vi "configuration UI.vi"() -> ()   [LabVIEW 2014, in "Tagbus PID Module editor node.lvclass"]
uses:
  Tagbus PID Module editor node.lvclass
  module/configuration/Tagbus PID Module configuration.lvclass
  <vilib>/NI/Module Execution Interface/Engine Configuration/engine configuration.lvclass
  <vilib>/NI/Tag Bus Data Framework/Configuration Editor/Classes/Module editor node/module editor node.lvclass
  <vilib>/NI/Tag Bus Data Framework/Configuration Editor/Classes/Engine Parent/Engine Parent Editor Node.lvclass
  <vilib>/NI/Configuration Framework/serializable configuration/NISE_CEF_serializable configuration.lvclass
  <vilib>/NI/Tag Bus Module Framework/channel/TBM channel.lvclass
  <vilib>/NI/Tools/Keyed Array/KeyedArray.ctl
  <vilib>/NI/Tools/Keyed Array/Tools_KeyedArray.lvlib
  <vilib>/NI/AMC/Message.ctl
  <vilib>/NI/AMC/AMC.lvlib
  <vilib>/NI/AMC/Message Queue.ctl
  <vilib>/NI/Configuration Framework/Node/NISE_CEF_Node.lvclass
  <vilib>/NI/Configuration Framework/Node/NodeRef.ctl
  <vilib>/NI/Configuration Framework/Controls/EventCluster.ctl
  <vilib>/NI/Configuration Framework/NISE_CEF_TreeControl.lvlib
  <vilib>/NI/Configuration Framework/Node/UserEventRef.ctl
  <vilib>/NI/Configuration Framework/Node/StopEvent.ctl
  <vilib>/NI/Configuration Framework/Node/RefreshUIEvent.ctl
  <vilib>/NI/Configuration Framework/Node/CacheState.ctl
  <vilib>/NI/Configuration Framework/Node/NodeChangeEvent.ctl
panel:
  in  "node change":T1
  in  "cache state":T2
  in  "refresh UI":T3
  in  "stop event":T4
  in  "Tab Control":enum32{"Static Configuration"}(tab)
  in  "hidden_remove":bool
  in  "hidden_settings":bool
  in  "hidden_Add":bool
  in  "Remove Button":bool
  in  "Add Button":bool
  in  "channel":i32(listbox)
  in  "settings":bool
  in  "user event":T5
  in  "main queue":T6
  in  "node ref":T7
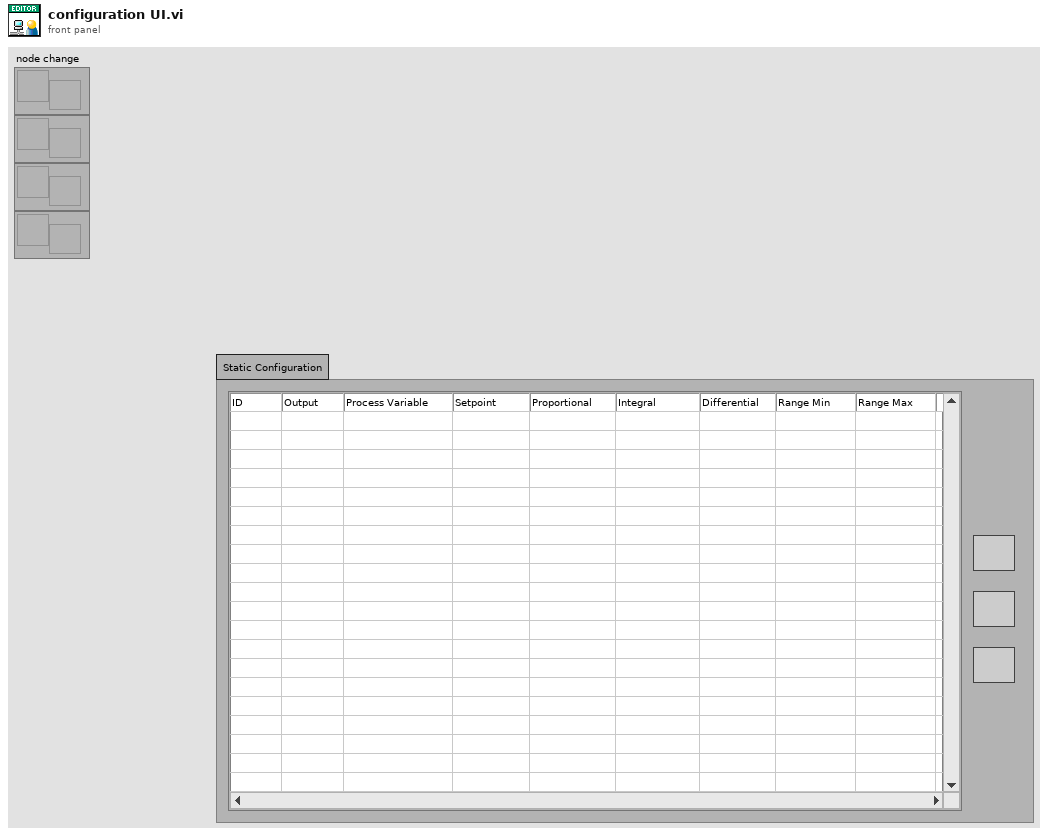
[diagram p1: front panel]
types:
  T1 = typedef "NISE_CEF_Node.lvclass/NodeChangeEvent.ctl" = refnum<user-event>
  T2 = typedef "NISE_CEF_Node.lvclass/CacheState.ctl" = refnum<user-event>
  T3 = typedef "NISE_CEF_Node.lvclass/RefreshUIEvent.ctl" = refnum<user-event>
  T4 = typedef "NISE_CEF_Node.lvclass/StopEvent.ctl" = refnum<user-event>
  T5 = typedef "NISE_CEF_Node.lvclass/UserEventRef.ctl" = refnum<user-event>
  T6 = typedef "AMC.lvlib/Message Queue.ctl" = refnum<queue>
  T7 = typedef "NISE_CEF_Node.lvclass/NodeRef.ctl" = refnum<data-value>
  T8 = typedef "Tagbus PID Module editor node.lvclass/table line.ctl" = cluster{"ID":string, "Setpoint":refnum<class "TBM channel.lvclass">, "Process Variable":refnum<class "TBM channel.lvclass">, "Output":refnum<class "TBM channel.lvclass">, "PID gains":cluster{"proportional gain (Kc)":dbl, "integral time (Ti, min)":dbl, "derivative time (Td, min)":dbl}, "output range":cluster{"output high":dbl, "output low":dbl}}
  T9 = cluster{"ID":string, "Setpoint":refnum<class "TBM channel.lvclass">, "Process Variable":refnum<class "TBM channel.lvclass">, "Output":refnum<class "TBM channel.lvclass">, "PID gains":cluster{"proportional gain (Kc)":dbl, "integral time (Ti, min)":dbl, "derivative time (Td, min)":dbl}, "output range":cluster{"output high":dbl, "output low":dbl}}
  T10 = typedef "LVPoint32TypeDef.ctl" = cluster{"Horizontal":i32, "Vertical":i32}
  T11 = typedef "LVRowAndColumnTypeDef.ctl" = cluster{"Row":i32, "Column":i32}
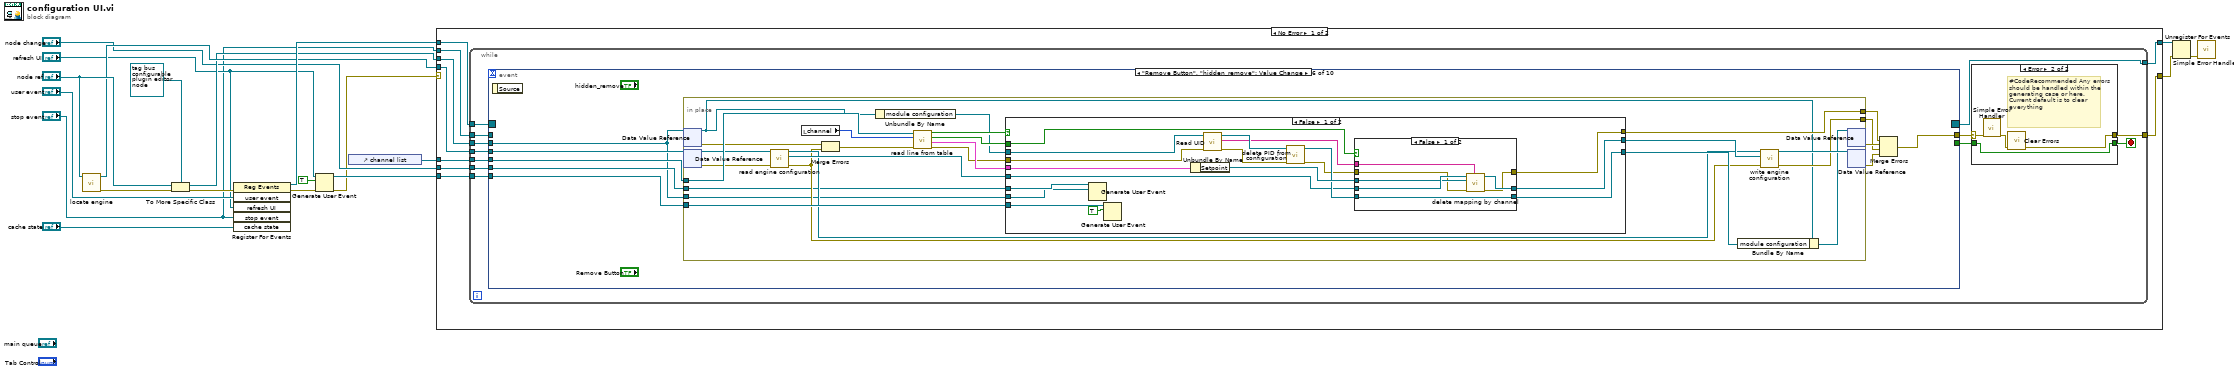
[diagram p0: block diagram]
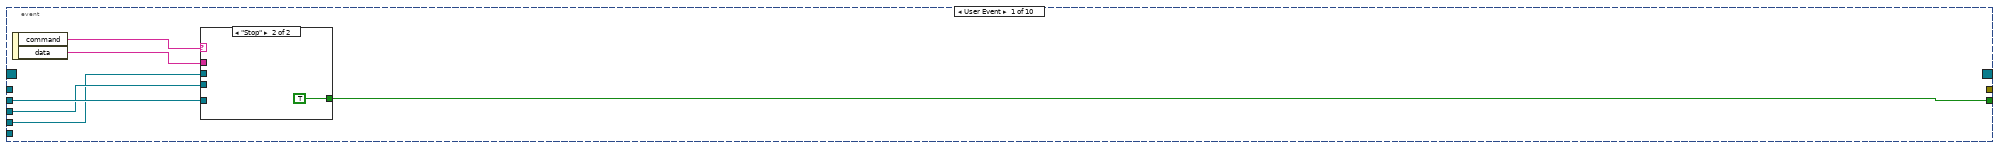
[diagram p3: hidden frame]
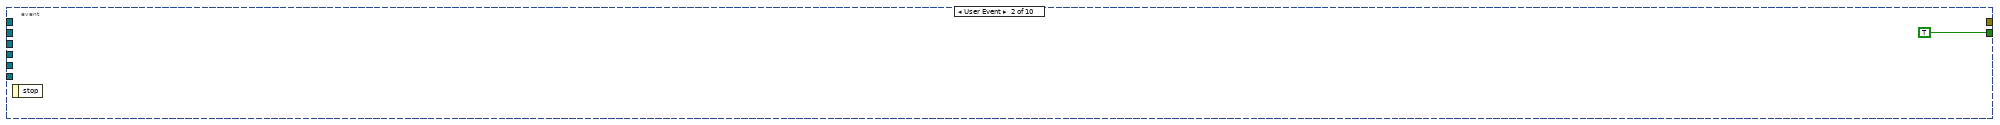
[diagram p5: hidden frame]
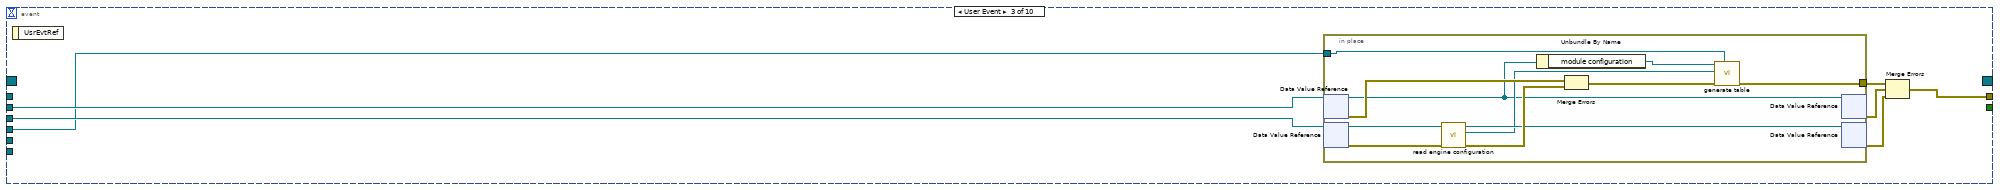
[diagram p6: hidden frame]
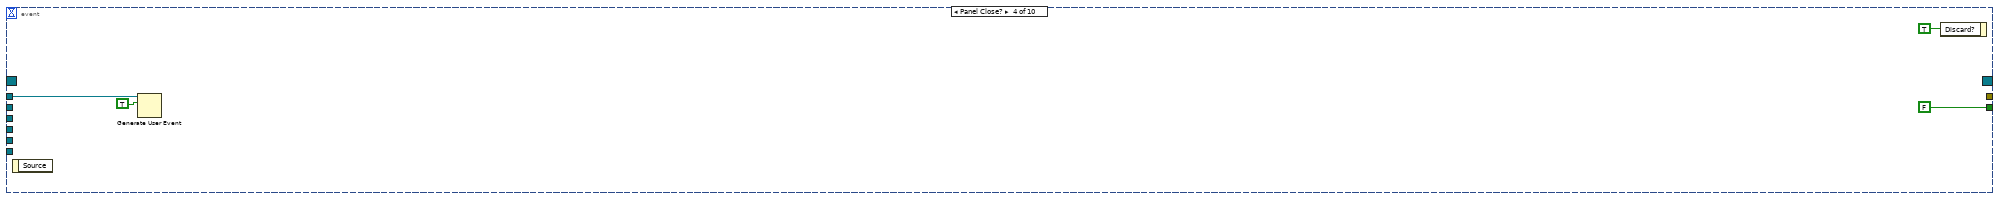
[diagram p7: hidden frame]
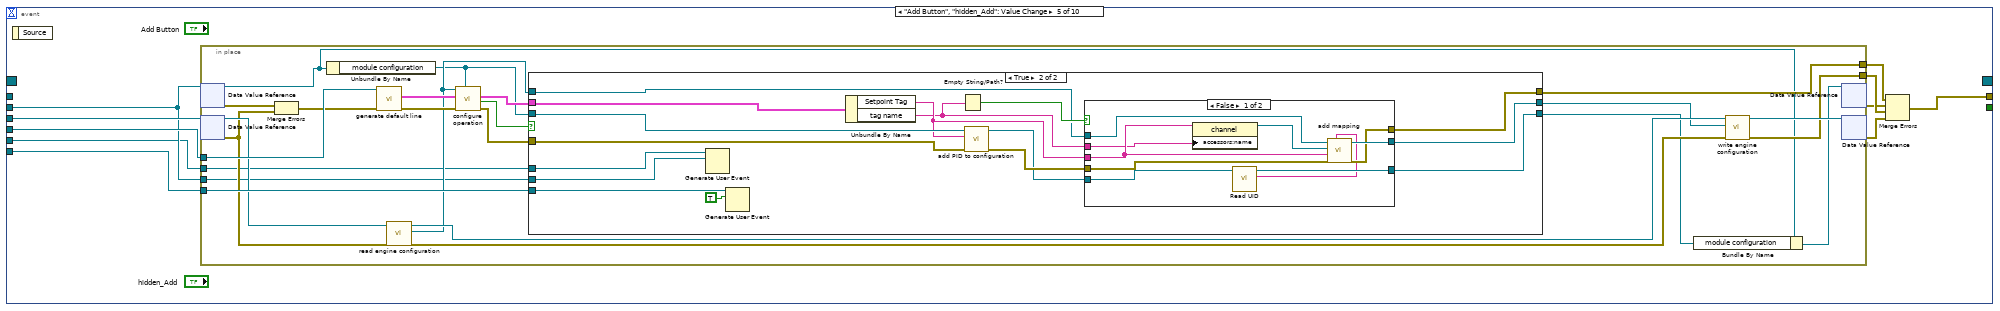
[diagram p8: hidden frame]
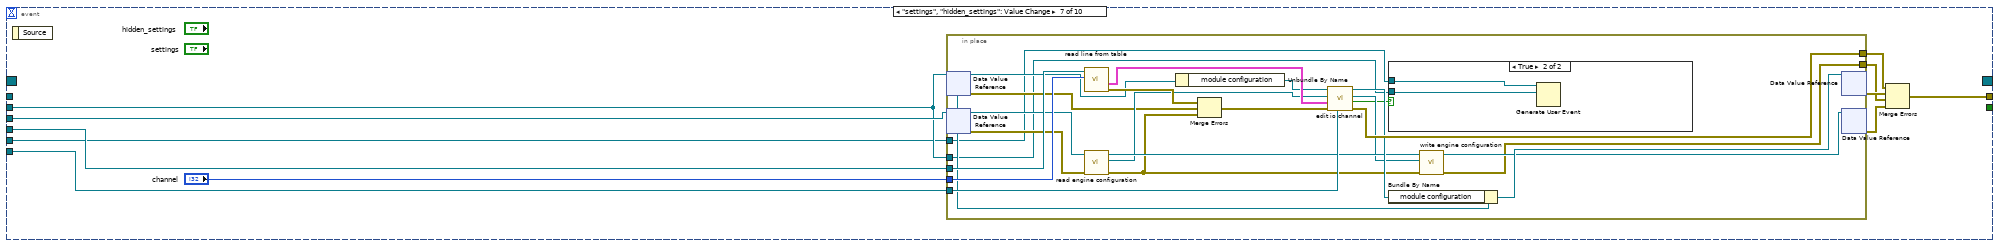
[diagram p13: hidden frame]
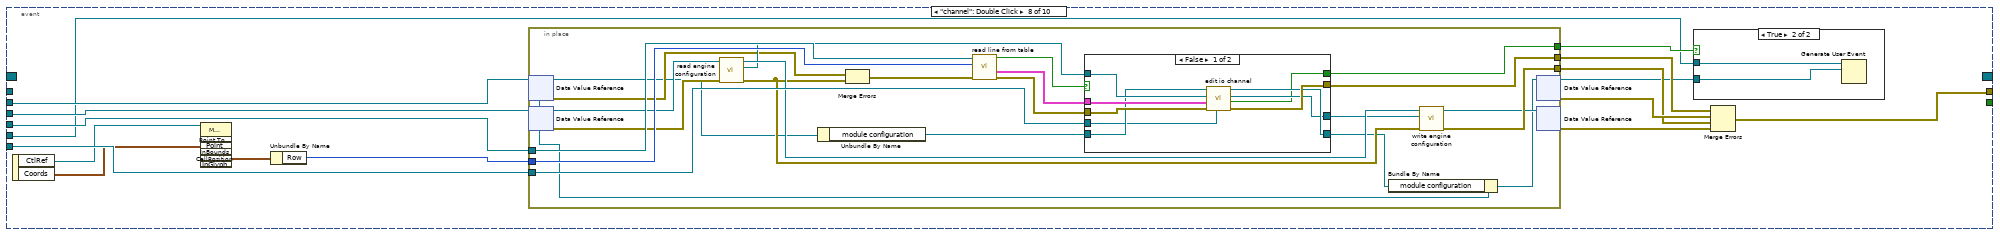
[diagram p15: hidden frame]
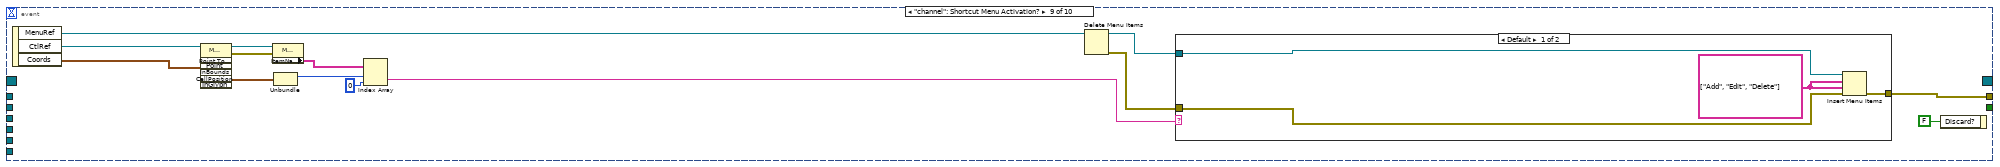
[diagram p18: hidden frame]
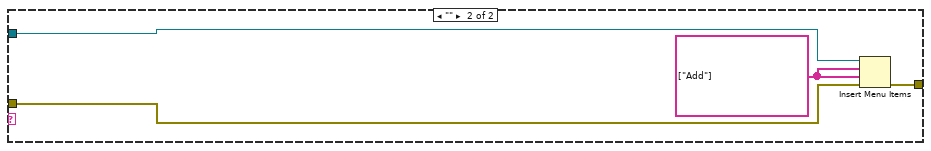
[diagram p19: hidden frame]
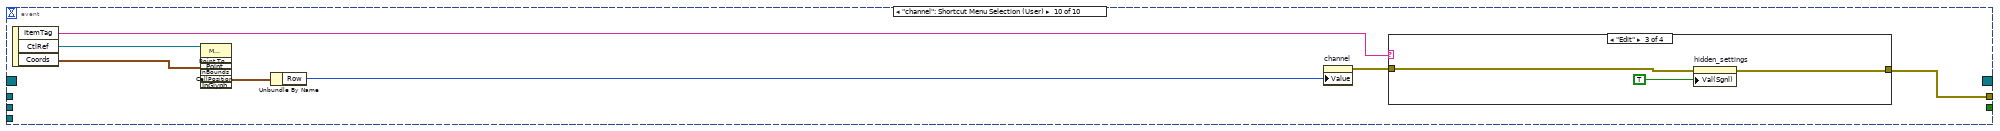
[diagram p20: hidden frame]
diagram:
  n1 = call <vilib>:"locate engine.vi"("component"="node ref") -> ("error out"=w8:errorcluster, "engine"=w15:refnum<data-value>)  [unwired: 9 in]
  n2 = To More Specific Class(target class=refnum<data-value> refnum ("data value reference"), reference="node ref", error in=w8) -> (specific class reference=w11:refnum<data-value>, error out=w10:errorcluster)
  n3 = register-events(error in=w10, "user event", "refresh UI", "stop event", "cache state") -> (reference out=w20:refnum<event-registration>, error out=w16:errorcluster)  [unwired: 1 in]
  n4 = Generate User Event(user event="refresh UI", event data cluster=TRUE ("event data"), error in=w16) -> (user event out=w7:T3, error out=w2:errorcluster)  [unwired: 1 in]
  n5 = control-ref of="channel list"() -> (w13:refnum<vi>)
  n6 = case shown="No Error" w2 {
    selector: w2 -> [_ w338]
    tunnel: w20 -> [w29 w337]
    tunnel: [w28 w337] -> w19
    tunnel: [w27 w338] -> w18
    tunnel: w15 -> [w26 _]
    tunnel: w13 -> [w25 _]
    tunnel: w11 -> [w24 _]
    tunnel: w7 -> [w23 _]
    tunnel: "node change" -> [w22 _]
    tunnel: "stop event" -> [w21 _]
    frame No Error {
      n7 = while {
        tunnel: w29 -> [w41]
        tunnel: [w40] -> w28
        tunnel: w24 -> [w36]
        tunnel: w26 -> [w35]
        tunnel: w23 -> [w34]
        tunnel: w25 -> [w32]
        tunnel: w22 -> [w31]
        tunnel: [w37] -> w27
        tunnel: w21 -> [w30]
        stop <- w39 stop-if-true
        n8 = event shown="[5] \"Remove Button\", \"hidden_remove\": Value Change" {
          selector: w41 -> [_ _ _ _ _ _ _ _ _ _]
          dyn-events: [_ _ _ _ _ _ _ _ _ _] -> w40
          timeout: _ -> [_ _ _ _ _ _ _ _ _ _]
          tunnel: [w53 TRUE _ FALSE _ _ _ _ _ _] -> w38
          tunnel: [_ _ w60 _ w84 w149 w216 w254 w298 w323] -> w33
          tunnel: w36 -> [w51 _ w62 _ w79 w144 w211 w250 _ _]
          tunnel: w35 -> [w50 _ w61 _ w83 w150 w215 w251 _ _]
          tunnel: w34 -> [_ _ _ _ w86 w152 w218 w260 _ _]
          tunnel: w32 -> [w48 _ w59 _ w85 w151 w217 w259 _ _]
          tunnel: w31 -> [_ _ _ _ w78 w145 w210 w246 _ _]
          tunnel: w30 -> [_ _ _ w75 _ _ _ _ _ _]
          event User Event {
            n9 = event-data() -> ("command"=w52:string, "data"=w49:string)  [unwired: 1 in]
            n10 = case shown="\"Stop\"" w52 {
              tunnel: [_ TRUE] -> w53
              tunnel: w51 -> [_ _]
              tunnel: w50 -> [_ _]
              tunnel: w49 -> [_ _]
              tunnel: w48 -> [_ _]
              frame Default {
              }
              frame "Stop" {
              }
            }
          }
          event User Event {
            n11 = event-data() -> ()  [unwired: 1 in, 1 out]
          }
          event User Event {
            n12 = event-data() -> ()  [unwired: 1 in, 1 out]
            n13 = in-place {
              in-place-border: [w73] -> w58
              in-place-border: w59 -> [w72]
              n14 = in-place-dvr #1(w62) -> (w64:refnum<class "Tagbus PID Module editor node.lvclass">, w70:errorcluster)
              n15 = in-place-dvr #2(w61) -> (w67:refnum<class "Engine Parent Editor Node.lvclass">, w69:errorcluster)
              n16 = call <vilib>:"read engine configuration.vi"("error in"=w69, "Engine Parent Editor Node in"=w67) -> ("error out"=w68:errorcluster, "engine configuration"=w65:refnum<class "engine configuration.lvclass">, "Engine Parent Editor Node out"=w66:refnum<class "Engine Parent Editor Node.lvclass">)  [unwired: 7 in]
              n17 = Unbundle By Name(w64) -> ("module configuration"=w63:refnum<class "Tagbus PID Module configuration.lvclass">)
              n18 = Merge Errors(w70, w68) -> (w71:errorcluster)
              n19 = call "generate table.vi"("table"=w72, "error in"=w71, "engine configuration"=w65, "tag bus configurable plugin module configuration"=w63) -> ("error out"=w73:errorcluster)  [unwired: 7 in]
              n20 = in-place-dvr #1(w64) -> (w57:errorcluster)  [unwired: 1 out]
              n21 = in-place-dvr #2(w66) -> (w56:errorcluster)  [unwired: 1 out]
            }
            n22 = Merge Errors(w58, w57, w56) -> (w60:errorcluster)
          }
          event Panel Close? {
            n23 = event-data() -> ()  [unwired: 1 in, 1 out]
            n24 = Generate User Event(user event=w75, event data cluster=TRUE ("event data")) -> ()  [unwired: 2 in, 2 out]
            n25 = event-data("Discard?"=TRUE) -> ()  [unwired: 1 in, 1 out]
          }
          event "Add Button", "hidden_Add": Value Change {
            n26 = event-data() -> ()  [unwired: 1 in, 1 out]
            n27 = in-place {
              in-place-border: [w111] -> w87
              in-place-border: w86 -> [w105]
              in-place-border: w85 -> [w104]
              in-place-border: [w99] -> w81
              in-place-border: w79 -> [w89]
              in-place-border: w78 -> [w88]
              n28 = in-place-dvr #3(w79) -> (w92:refnum<class "Tagbus PID Module editor node.lvclass">, w93:errorcluster)
              n29 = in-place-dvr #4(w83) -> (w102:refnum<class "Engine Parent Editor Node.lvclass">, w101:errorcluster)
              n30 = Merge Errors(w93, w101) -> (w103:errorcluster)
              n31 = Unbundle By Name(w92) -> ("module configuration"=w94:refnum<class "Tagbus PID Module configuration.lvclass">)
              n32 = call "generate default line.vi"("error in"=w103, "operations table"=w104) -> ("error out"=w109:errorcluster, "line"=w110:T8)  [unwired: 8 in]
              n33 = call <vilib>:"read engine configuration.vi"("error in"=w101, "Engine Parent Editor Node in"=w102) -> ("error out"=w97:errorcluster, "engine configuration"=w95:refnum<class "engine configuration.lvclass">, "Engine Parent Editor Node out"=w98:refnum<class "Engine Parent Editor Node.lvclass">)  [unwired: 7 in]
              n34 = call "configure operation.vi"("tag bus configurable plugin module configuration"=w94, "error in"=w109, "line item in"=w110, "engine configuration"=w95) -> ("error out"=w107:errorcluster, "success"=w106:bool, "line item out"=w108:T8)  [unwired: 4 in, 1 out]
              n35 = case shown="True" w106 {
                tunnel: [w114 w119] -> w111
                tunnel: w107 -> [w114 w128]
                tunnel: w95 -> [w113 w126]
                tunnel: w108 -> [_ w129]
                tunnel: w94 -> [w112 w130]
                tunnel: [w113 w125] -> w96
                tunnel: [w112 w120] -> w91
                tunnel: w105 -> [_ w118]
                tunnel: w89 -> [_ w116]
                tunnel: w88 -> [_ w115]
                frame False {
                }
                frame True {
                  n36 = Generate User Event(user event=w115, event data cluster=w116) -> ()  [unwired: 2 in, 2 out]
                  n37 = Generate User Event(user event=w118, event data cluster=TRUE ("event data")) -> ()  [unwired: 2 in, 2 out]
                  n38 = Unbundle By Name(w129) -> ("Setpoint Tag"=w123:string, "tag name"=w122:string)
                  n39 = Empty String/Path?(string/path=w122) -> (empty?=w127:bool)
                  n40 = call "add PID to configuration.vi"("error in"=w128, "PID in"=w123, "Tagbus PID Module configuration in"=w130) -> ("error out"=w124:errorcluster, "Tagbus PID Module configuration out"=w121:refnum<class "Tagbus PID Module configuration.lvclass">)  [unwired: 7 in]
                  n41 = case shown="False" w127 {
                    tunnel: w126 -> [w140 w143]
                    tunnel: [w139 w143] -> w125
                    tunnel: w124 -> [w138 w142]
                    tunnel: w123 -> [w137 _]
                    tunnel: w122 -> [w136 _]
                    tunnel: [w134 w142] -> w119
                    tunnel: w121 -> [w133 w141]
                    tunnel: [w132 w141] -> w120
                    frame False {
                      n42 = property class="channel"(reference=w137, "accessors:name"=w136) -> (reference out=w135:refnum<class "TBM channel.lvclass">)  [unwired: 1 in, 1 out]
                      n43 = call <vilib>:"Read UID.vi"("configuration in"=w133) -> ("instance id"=w131:string, "configuration out"=w132:refnum<class "Tagbus PID Module configuration.lvclass">)  [unwired: 8 in, 1 out]
                      n44 = call <vilib>:"add mapping.vi"("owner ID"=w131, "error in"=w138, "channel"=w137, "tag descriptor"=w135, "engine configuration"=w140) -> ("error out"=w134:errorcluster, "engine configuration out"=w139:refnum<class "engine configuration.lvclass">)  [unwired: 5 in]
                    }
                    frame True {
                    }
                  }
                }
              }
              n45 = Bundle By Name(cluster=w92, "module configuration"=w91) -> (w90:refnum<class "Tagbus PID Module editor node.lvclass">)
              n46 = call <vilib>:"write engine configuration.vi"("error in"=w97, "engine configuration"=w96, "Engine Parent Editor Node in"=w98) -> ("error out"=w99:errorcluster, "Engine Parent Editor Node out"=w100:refnum<class "Engine Parent Editor Node.lvclass">)  [unwired: 7 in]
              n47 = in-place-dvr #3(w90) -> (w80:errorcluster)  [unwired: 1 out]
              n48 = in-place-dvr #4(w100) -> (w82:errorcluster)  [unwired: 1 out]
            }
            n49 = Merge Errors(w87, w80, w81, w82) -> (w84:errorcluster)
          }
          event "Remove Button", "hidden_remove": Value Change {
            n50 = event-data() -> ()  [unwired: 1 in, 1 out]
            n51 = in-place {
              in-place-border: [w177] -> w153
              in-place-border: w152 -> [w171]
              in-place-border: w151 -> [w170]
              in-place-border: [w168] -> w146
              in-place-border: w145 -> [w155]
              in-place-border: w144 -> [w154]
              n52 = in-place-dvr #5(w144) -> (w161:refnum<class "Tagbus PID Module editor node.lvclass">, w156:errorcluster)
              n53 = in-place-dvr #6(w150) -> (w164:refnum<class "Engine Parent Editor Node.lvclass">, w163:errorcluster)
              n54 = call <vilib>:"read engine configuration.vi"("error in"=w163, "Engine Parent Editor Node in"=w164) -> ("error out"=w157:errorcluster, "engine configuration"=w159:refnum<class "engine configuration.lvclass">, "Engine Parent Editor Node out"=w158:refnum<class "Engine Parent Editor Node.lvclass">)  [unwired: 7 in]
              n55 = local read "channel"() -> (w176:i32)
              n56 = Merge Errors(w156, w157) -> (w162:errorcluster)
              n57 = Unbundle By Name(w161) -> ("module configuration"=w160:refnum<class "Tagbus PID Module configuration.lvclass">)
              n58 = call "read line from table.vi"("error in"=w162, "line number"=w176, "channels table"=w170) -> ("error out"=w172:errorcluster, "line"=w175:T8, "empty tag?"=w173:bool, "empty channel?"=w174:bool)  [unwired: 5 in]
              n59 = case shown="False" w174 {
                tunnel: [w187 w208] -> w177
                tunnel: w175 -> [w196 _]
                tunnel: w160 -> [w184 w207]
                tunnel: w159 -> [w190 w209]
                tunnel: w173 -> [w195 _]
                tunnel: w172 -> [w193 w208]
                tunnel: [w189 w209] -> w165
                tunnel: [w188 w207] -> w166
                tunnel: w171 -> [w186 _]
                tunnel: w155 -> [w181 _]
                tunnel: w154 -> [w180 _]
                frame False {
                  n60 = Generate User Event(user event=w181, event data cluster=w180) -> ()  [unwired: 2 in, 2 out]
                  n61 = Generate User Event(user event=w186, event data cluster=TRUE ("event data")) -> ()  [unwired: 2 in, 2 out]
                  n62 = Unbundle By Name(w196) -> ("Setpoint"=w194:refnum<class "TBM channel.lvclass">)
                  n63 = call <vilib>:"Read UID.vi"("error in"=w193, "configuration in"=w184) -> ("error out"=w185:errorcluster, "instance id"=w182:string, "configuration out"=w183:refnum<class "Tagbus PID Module configuration.lvclass">)  [unwired: 7 in]
                  n64 = call "delete PID from configuration.vi"("error in"=w185, "Tagbus PID Module configuration in"=w183) -> ("error out"=w191:errorcluster, "Tagbus PID Module configuration out"=w192:refnum<class "Tagbus PID Module configuration.lvclass">, "PID In"=w178:T9)  [unwired: 7 in]
                  n65 = case shown="False" w195 {
                    tunnel: w194 -> [w202 _]
                    tunnel: w192 -> [w198 w204]
                    tunnel: w191 -> [w201 w205]
                    tunnel: w190 -> [w203 w206]
                    tunnel: [w200 w206] -> w189
                    tunnel: [w199 w205] -> w187
                    tunnel: [w198 w204] -> w188
                    tunnel: w182 -> [w197 _]
                    frame False {
                      n66 = call <vilib>:"delete mapping by channel.vi"("owner ID"=w197, "error in"=w201, "channel"=w202, "engine configuration in"=w203) -> ("error out"=w199:errorcluster, "engine configuration out"=w200:refnum<class "engine configuration.lvclass">)  [unwired: 6 in]
                    }
                    frame True {
                    }
                  }
                }
                frame True {
                }
              }
              n67 = Bundle By Name(cluster=w161, "module configuration"=w166) -> (w167:refnum<class "Tagbus PID Module editor node.lvclass">)
              n68 = call <vilib>:"write engine configuration.vi"("error in"=w157, "engine configuration"=w165, "Engine Parent Editor Node in"=w158) -> ("error out"=w168:errorcluster, "Engine Parent Editor Node out"=w169:refnum<class "Engine Parent Editor Node.lvclass">)  [unwired: 7 in]
              n69 = in-place-dvr #5(w167) -> (w147:errorcluster)  [unwired: 1 out]
              n70 = in-place-dvr #6(w169) -> (w148:errorcluster)  [unwired: 1 out]
            }
            n71 = Merge Errors(w153, w147, w146, w148) -> (w149:errorcluster)
          }
          event "settings", "hidden_settings": Value Change {
            n72 = event-data() -> ()  [unwired: 1 in, 1 out]
            n73 = in-place {
              in-place-border: [w243] -> w220
              in-place-border: "channel" -> [w240]
              in-place-border: w218 -> [w239]
              in-place-border: w217 -> [w238]
              in-place-border: [w231] -> w212
              in-place-border: w211 -> [w222]
              in-place-border: w210 -> [w221]
              n74 = in-place-dvr #7(w211) -> (w237:refnum<class "Tagbus PID Module editor node.lvclass">, w224:errorcluster)
              n75 = in-place-dvr #8(w215) -> (w234:refnum<class "Engine Parent Editor Node.lvclass">, w233:errorcluster)
              n76 = call "read line from table.vi"("line number"=w240, "channels table"=w238) -> ("error out"=w242:errorcluster, "line"=w241:T8)  [unwired: 6 in, 2 out]
              n77 = call <vilib>:"read engine configuration.vi"("error in"=w233, "Engine Parent Editor Node in"=w234) -> ("error out"=w225:errorcluster, "engine configuration"=w227:refnum<class "engine configuration.lvclass">, "Engine Parent Editor Node out"=w229:refnum<class "Engine Parent Editor Node.lvclass">)  [unwired: 7 in]
              n78 = Unbundle By Name(w237) -> ("module configuration"=w230:refnum<class "Tagbus PID Module configuration.lvclass">)
              n79 = Merge Errors(w242, w224, w225) -> (w226:errorcluster)
              n80 = call "edit io channel.vi"("refresh UI"=w239, "error in"=w226, "line"=w241, "engine configuration in"=w227, "tag bus configurable plugin module configuration in"=w230) -> ("error out"=w243:errorcluster, "change?"=w223:bool, "engine configuration"=w228:refnum<class "engine configuration.lvclass">, "tag bus configurable plugin module configuration out"=w235:refnum<class "Tagbus PID Module configuration.lvclass">)  [unwired: 3 in]
              n81 = case shown="True" w223 {
                tunnel: w222 -> [_ w245]
                tunnel: w221 -> [_ w244]
                frame False {
                }
                frame True {
                  n82 = Generate User Event(user event=w244, event data cluster=w245) -> ()  [unwired: 2 in, 2 out]
                }
              }
              n83 = Bundle By Name(cluster=w237, "module configuration"=w235) -> (w236:refnum<class "Tagbus PID Module editor node.lvclass">)
              n84 = call <vilib>:"write engine configuration.vi"("error in"=w225, "engine configuration"=w228, "Engine Parent Editor Node in"=w229) -> ("error out"=w231:errorcluster, "Engine Parent Editor Node out"=w232:refnum<class "Engine Parent Editor Node.lvclass">)  [unwired: 7 in]
              n85 = in-place-dvr #7(w236) -> (w213:errorcluster)  [unwired: 1 out]
              n86 = in-place-dvr #8(w232) -> (w214:errorcluster)  [unwired: 1 out]
            }
            n87 = Merge Errors(w220, w213, w212, w214) -> (w216:errorcluster)
          }
          event "channel": Double Click {
            n88 = event-data() -> ("CtlRef"=w258:refnum<vi>, "Coords"=w257:T10)  [unwired: 1 in]
            n89 = invoke class="MCListbox (strict)" method="Point To Row Column"(reference=w258, "Point"=w257) -> ("CellPosition"=w256:T11)  [unwired: 5 in, 6 out]
            n90 = Unbundle By Name(w256) -> ("Row"=w255:i32)
            n91 = in-place {
              in-place-border: [w285] -> w261
              in-place-border: w260 -> [w282]
              in-place-border: w259 -> [w281]
              in-place-border: w255 -> [w280]
              in-place-border: [w277] -> w249
              in-place-border: [w264] -> w248
              n92 = in-place-dvr #9(w250) -> (w266:refnum<class "Tagbus PID Module editor node.lvclass">, w271:errorcluster)
              n93 = in-place-dvr #10(w251) -> (w275:refnum<class "Engine Parent Editor Node.lvclass">, w274:errorcluster)
              n94 = call <vilib>:"read engine configuration.vi"("error in"=w274, "Engine Parent Editor Node in"=w275) -> ("error out"=w270:errorcluster, "engine configuration"=w272:refnum<class "engine configuration.lvclass">, "Engine Parent Editor Node out"=w273:refnum<class "Engine Parent Editor Node.lvclass">)  [unwired: 7 in]
              n95 = Unbundle By Name(w266) -> ("module configuration"=w265:refnum<class "Tagbus PID Module configuration.lvclass">)
              n96 = Merge Errors(w271, w270) -> (w278:errorcluster)
              n97 = call "read line from table.vi"("error in"=w278, "line number"=w280, "channels table"=w281) -> ("error out"=w284:errorcluster, "line"=w283:T8, "empty channel?"=w279:bool)  [unwired: 5 in, 1 out]
              n98 = case shown="False" w279 {
                tunnel: [w294 w295] -> w285
                tunnel: w284 -> [w293 w295]
                tunnel: w283 -> [w292 _]
                tunnel: w272 -> [w291 w296]
                tunnel: w265 -> [w290 w297]
                tunnel: [w289 w297] -> w268
                tunnel: [w288 w296] -> w269
                tunnel: w282 -> [w287 _]
                tunnel: [w286 _] -> w264
                frame False {
                  n99 = call "edit io channel.vi"("refresh UI"=w287, "error in"=w293, "line"=w292, "engine configuration in"=w291, "tag bus configurable plugin module configuration in"=w290) -> ("error out"=w294:errorcluster, "change?"=w286:bool, "engine configuration"=w288:refnum<class "engine configuration.lvclass">, "tag bus configurable plugin module configuration out"=w289:refnum<class "Tagbus PID Module configuration.lvclass">)  [unwired: 3 in]
                }
                frame True {
                }
              }
              n100 = Bundle By Name(cluster=w266, "module configuration"=w268) -> (w267:refnum<class "Tagbus PID Module editor node.lvclass">)
              n101 = call <vilib>:"write engine configuration.vi"("error in"=w270, "engine configuration"=w269, "Engine Parent Editor Node in"=w273) -> ("error out"=w277:errorcluster, "Engine Parent Editor Node out"=w276:refnum<class "Engine Parent Editor Node.lvclass">)  [unwired: 7 in]
              n102 = in-place-dvr #9(w267) -> (w247:refnum<data-value>, w252:errorcluster)
              n103 = in-place-dvr #10(w276) -> (w253:errorcluster)  [unwired: 1 out]
            }
            n104 = case shown="True" w248 {
              tunnel: w247 -> [_ w263]
              tunnel: w246 -> [_ w262]
              frame False {
              }
              frame True {
                n105 = Generate User Event(user event=w262, event data cluster=w263) -> ()  [unwired: 2 in, 2 out]
              }
            }
            n106 = Merge Errors(w261, w252, w249, w253) -> (w254:errorcluster)
          }
          event "channel": Shortcut Menu Activation? {
            n107 = event-data() -> ("MenuRef"=w308:refnum<k9>, "CtlRef"=w310:refnum<vi>, "Coords"=w309:T10)  [unwired: 1 in]
            n108 = invoke class="MCListbox (strict)" method="Point To Row Column"(reference=w310, "Point"=w309) -> (reference out=w307:refnum<vi>, error out=w306:errorcluster, "CellPosition"=w305:T11)  [unwired: 5 in, 4 out]
            n109 = property class="MCListbox (strict)"(reference=w307, error in=w306) -> ("ItemNames"=w304:string[][])  [unwired: 2 out]
            n110 = Unbundle(w305) -> ("Row"=w303:i32)  [unwired: 1 out]
            n111 = Index Array(array=w304, index (row)=w303, index (col)=0 ("disabled index (col)")) -> (element=w301:string)
            n112 = Delete Menu Items(9:w308) -> (0:w299:errorcluster, 3:w300:refnum<k9>)  [unwired: 3 in]
            n113 = case shown="Default" w301 {
              tunnel: w300 -> [w315 w319]
              tunnel: w299 -> [w314 w318]
              tunnel: [w313 w317] -> w298
              frame Default {
                w312 = string[] ["Add", "Edit", "Delete"] ("item names")
                n114 = Insert Menu Items(6:w314, 7:w312, 8:w312, 9:w315) -> (0:w313:errorcluster)  [unwired: 2 in, 2 out]
              }
              frame "" {
                w316 = string[] ["Add"] ("item names")
                n115 = Insert Menu Items(6:w318, 7:w316, 8:w316, 9:w319) -> (0:w317:errorcluster)  [unwired: 2 in, 2 out]
              }
            }
            n116 = event-data("Discard?"=FALSE) -> ()  [unwired: 1 in, 1 out]
          }
          event "channel": Shortcut Menu Selection (User) {
            n117 = event-data() -> ("ItemTag"=w324:string, "CtlRef"=w325:refnum<vi>, "Coords"=w326:T10)  [unwired: 1 in]
            n118 = invoke class="MCListbox (strict)" method="Point To Row Column"(reference=w325, "Point"=w326) -> ("CellPosition"=w321:T11)  [unwired: 5 in, 6 out]
            n119 = Unbundle By Name(w321) -> ("Row"=w320:i32)
            n120 = property on="channel" class="MCListbox (strict)"("Value"=w320) -> (error out=w322:errorcluster)  [unwired: 2 in, 1 out]
            n121 = case shown="\"Edit\"" w324 {
              tunnel: w322 -> [w327 w329 w333 w336]
              tunnel: [w327 w328 w332 w335] -> w323
              frame Default {
              }
              frame "Add" {
                n122 = property on="hidden_Add" class="Bool (strict)"(error in=w329, "Val(Sgnl)"=TRUE ("Value (Signaling)")) -> (error out=w328:errorcluster)  [unwired: 1 in, 1 out]
              }
              frame "Edit" {
                n123 = property on="hidden_settings" class="Bool (strict)"(error in=w333, "Val(Sgnl)"=TRUE ("Value (Signaling)")) -> (error out=w332:errorcluster)  [unwired: 1 in, 1 out]
              }
              frame "Delete" {
                n124 = property on="hidden_remove" class="Bool (strict)"(error in=w336, "Val(Sgnl)"=FALSE ("Value (Signaling)")) -> (error out=w335:errorcluster)  [unwired: 1 in, 1 out]
              }
            }
          }
        }
        n125 = case shown="Error" w33 {
          selector: w33 -> [w42 w46]
          tunnel: [w43 w47] -> w39
          tunnel: w38 -> [w43 w47]
          tunnel: [w42 w44] -> w37
          frame No Error {
          }
          frame Error {
            # "#CodeRecommended Any errors should be handled within the generating case or here. Current default is to clear everything"
            n126 = call <vilib>:"Simple Error Handler.vi"("error in (no error)"=w46) -> ("error out"=w45:errorcluster)  [unwired: 4 in, 4 out]
            n127 = call <vilib>:"Clear Errors.vi"("error in (no error)"=w45) -> ("error out"=w44:errorcluster)  [unwired: 5 in, 1 out]
          }
        }
      }
    }
    frame Error {
    }
  }
  n128 = Unregister For Events(event registration refnum=w19, error in=w18) -> (error out=w14:errorcluster)
  n129 = call <vilib>:"Simple Error Handler.vi"("error in (no error)"=w14) -> ()  [unwired: 4 in, 5 out]
